vi "Beverage_Create.vi"(0 "reference in":refnum<class "Beverage.lvclass">, 2 "Description":string="Not defined", 5 "error in (no error)":errorcluster) -> (14 "reference out":refnum<class "Beverage.lvclass">, 19 "error out":errorcluster)   [LabVIEW 2020, in "Beverage.lvclass"]
doc: "This VI initializes the attribute \"Description\" that is inherited from concrete type of beverages."
uses:
  Beverage.lvclass
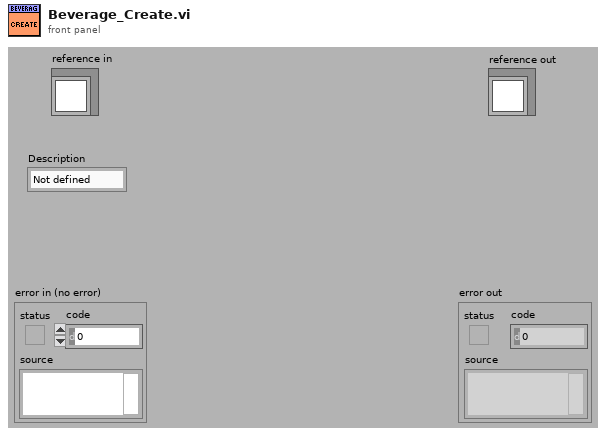
[diagram p1: front panel]
types:
  T1 = typedef "Beverage.lvclass/ObjectAttributes.ctl" = cluster{"Description":string}
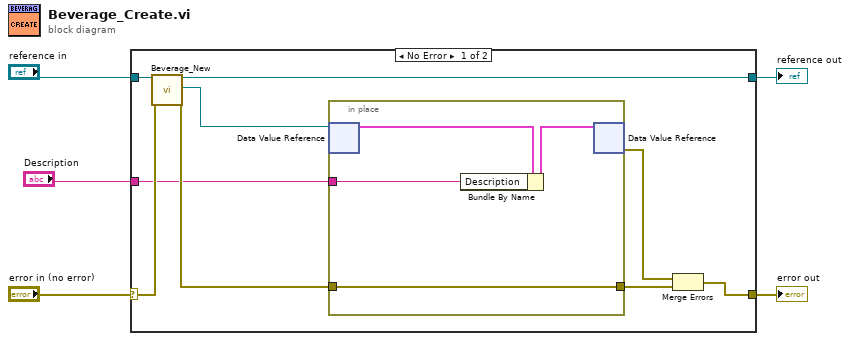
[diagram p0: block diagram]
diagram:
  n1 = case shown="No Error" "error in (no error)" {
    selector: "error in (no error)" -> [w13 w20]
    tunnel: [w10 w20] -> w4
    tunnel: "reference in" -> [w14 w19]
    tunnel: [w12 w19] -> w2
    tunnel: "Description" -> [w6 _]
    frame No Error {
      n2 = call "Beverage_New.vi"("reference in"=w14, "error in (no error)"=w13) -> ("reference out"=w12:refnum<class "Beverage.lvclass">, "DVRRefOut"=w9:refnum<data-value>, "error out"=w8:errorcluster)  [unwired: 14 in, 1 out]
      n3 = in-place {
        in-place-border: w8 -> [w16]
        in-place-border: [w16] -> w7
        in-place-border: w6 -> [w15]
        n4 = in-place-dvr #1(w9) -> (w17:T1)  [unwired: 1 out]
        n5 = Bundle By Name(cluster=w17, "Description"=w15) -> (w18:T1)
        n6 = in-place-dvr #1(w18) -> (w11:errorcluster)  [unwired: 1 out]
      }
      n7 = Merge Errors(w11, w7) -> (w10:errorcluster)
    }
    frame Error {
    }
  }
  "error out" <- w4
  "reference out" <- w2
